vi "GoToField.vi"(8 "error in (no error)":errorcluster, 9 "Target Field Rate (T/min)":dbl, 10 "Target Field (T)":dbl, 11 "Magnet in":refnum<class "Magnet.lvclass">) -> (0 "error out":errorcluster, 3 "Magnet out":refnum<class "Magnet.lvclass">)   [LabVIEW 2016, in "Magnet.lvclass"]
uses:
  Magnet.lvclass
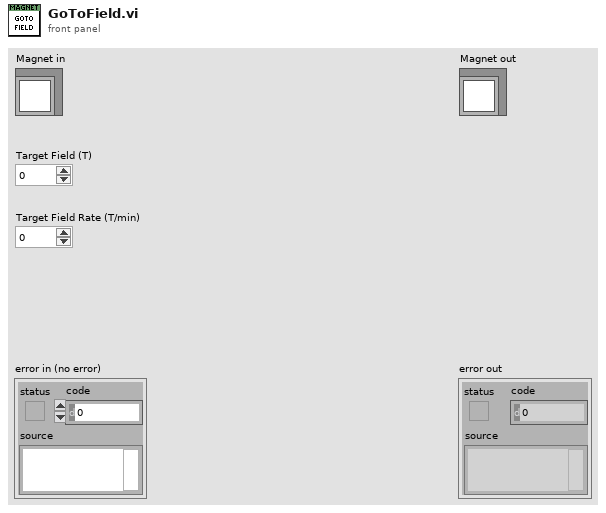
[diagram p1: front panel]
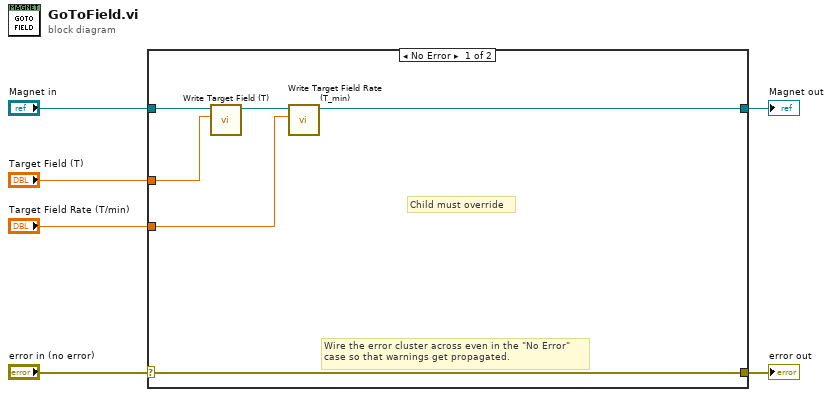
[diagram p0: block diagram]
diagram:
  n1 = case shown="No Error" "error in (no error)" {
    selector: "error in (no error)" -> [w12 w14]
    tunnel: [w12 w14] -> w5
    tunnel: [w9 w13] -> w3
    tunnel: "Magnet in" -> [w10 w13]
    tunnel: "Target Field Rate (T/min)" -> [w8 _]
    tunnel: "Target Field (T)" -> [w7 _]
    frame No Error {
      # "Child must override"
      # "Wire the error cluster across even in the \"No Error\"\ncase so that warnings get propagated."
      n2 = call-dynamic "Write Target Field (T).vi"("Target Field (T)"=w7, "Magnet in"=w10) -> ("Magnet out"=w11:refnum<class "Magnet.lvclass">)  [unwired: 8 in, 1 out]
      n3 = call-dynamic "Write Target Field Rate (T_min).vi"("Target Field Rate (T/min)"=w8, "Magnet in"=w11) -> ("Magnet out"=w9:refnum<class "Magnet.lvclass">)  [unwired: 8 in, 1 out]
    }
    frame Error {
    }
  }
  "error out" <- w5
  "Magnet out" <- w3
